vi "RSNRPZ Get Device Info Z5.vi"(8 "error in (no error)":errorcluster, 9 "Port (A)":i32(ring) items=["A", "B", "C", "D"], 11 "VISA session":refnum<visa-resource-name> caption="VISA resource name") -> (0 "error out":errorcluster, 1 "Sensor Type":string, 2 "Sensor Name":string, 3 "dup VISA session":refnum<visa-resource-name> caption="VISA resource name", 4 "Sensor Serial":string, 5 "Connected":bool)   [LabVIEW 2010]
doc: "If the above status VI (= NrpGetDeviceStatusZ5() ) indicates that there is an NRP-Z5, this VI supplies information about the connected devices at its ports A...D (using 'iPortIdx' = 0...3)."
uses:
  rsnrpz_32.dll
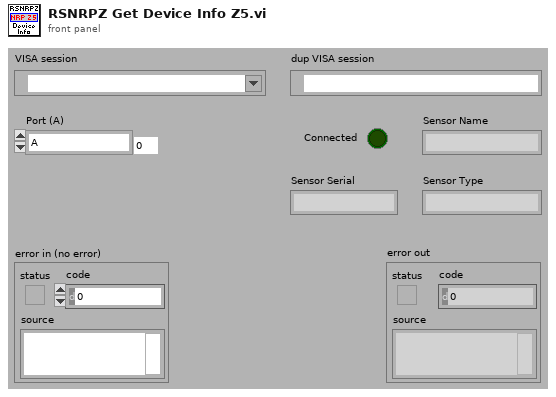
[diagram p1: front panel]
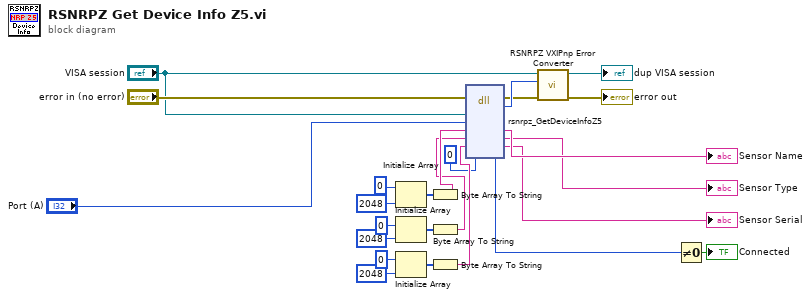
[diagram p0: block diagram]
diagram:
  n1 = Initialize Array(u8 0 ("element"), 2048 ("dimension size")) -> (w17:u8[])
  n2 = Initialize Array(u8 0 ("element"), 2048 ("dimension size")) -> (w13:u8[])
  n3 = Initialize Array(u8 0 ("element"), 2048 ("dimension size")) -> (w9:u8[])
  n4 = Byte Array To String(unsigned byte array=w17) -> (string=w18:string)
  n5 = Byte Array To String(unsigned byte array=w13) -> (string=w14:string)
  n6 = Byte Array To String(unsigned byte array=w9) -> (string=w10:string)
  n7 = dll-call lib="rsnrpz_32.dll" fn="rsnrpz_GetDeviceInfoZ5"(error in="error in (no error)", "Instrument Handle"="VISA session", "Port"="Port (A)", "Sensor Name"=w18, "Sensor Type"=w14, "Sensor Serial"=w10, "Connected"=i16 0) -> (error out=w5:errorcluster, w19:i32, "Sensor Name"=→"Sensor Name":string, "Sensor Type"=→"Sensor Type":string, "Sensor Serial"=→"Sensor Serial":string, "Connected"=w20:i16)  [unwired: 4 in, 1 out]
  n8 = call <instrlib>:"RSNRPZ VXIPnp Error Converter.vi"("error in"=w5, "VXIPnp error code"=w19, "VISA session"="VISA session") -> ("error out"=→"error out":errorcluster, "dup VISA session"=→"dup VISA session":refnum<visa-resource-name>)  [unwired: 7 in]
  n9 = Not Equal To 0?(x=w20) -> (x != 0?=→"Connected":bool)
